vi "st_Wilcoxon diff test.vi"(6 "alternative hypothesis":i32(ring) items=["mean(pop) != mean"=0, "mean(pop) > mean"=1, "mean(pop) < mean"=-1], 9 "significance level":dbl=0.05, 11 "Xi - Yi":dbl[](array[numeric])) -> (0 "error":i32, 2 "p value":dbl, 3 "reject the null hypothesis":bool)   [LabVIEW 2020, in "NI_Gmath.lvlib"]
uses:
  NI_Gmath.lvlib
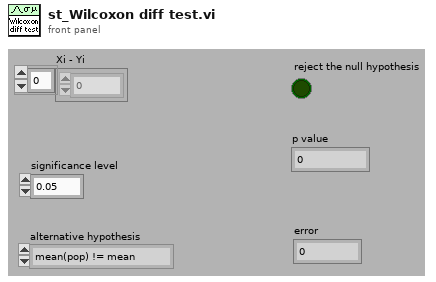
[diagram p1: front panel]
types:
  T1 = cluster{"n":u8, "x min":u8, "x max":u8, "P{W+ >= x}":sgl[]}[]
  T2 = cluster{"n":u8, "x min":u8, "x max":u8, "P{W+ >= x}":sgl[]}
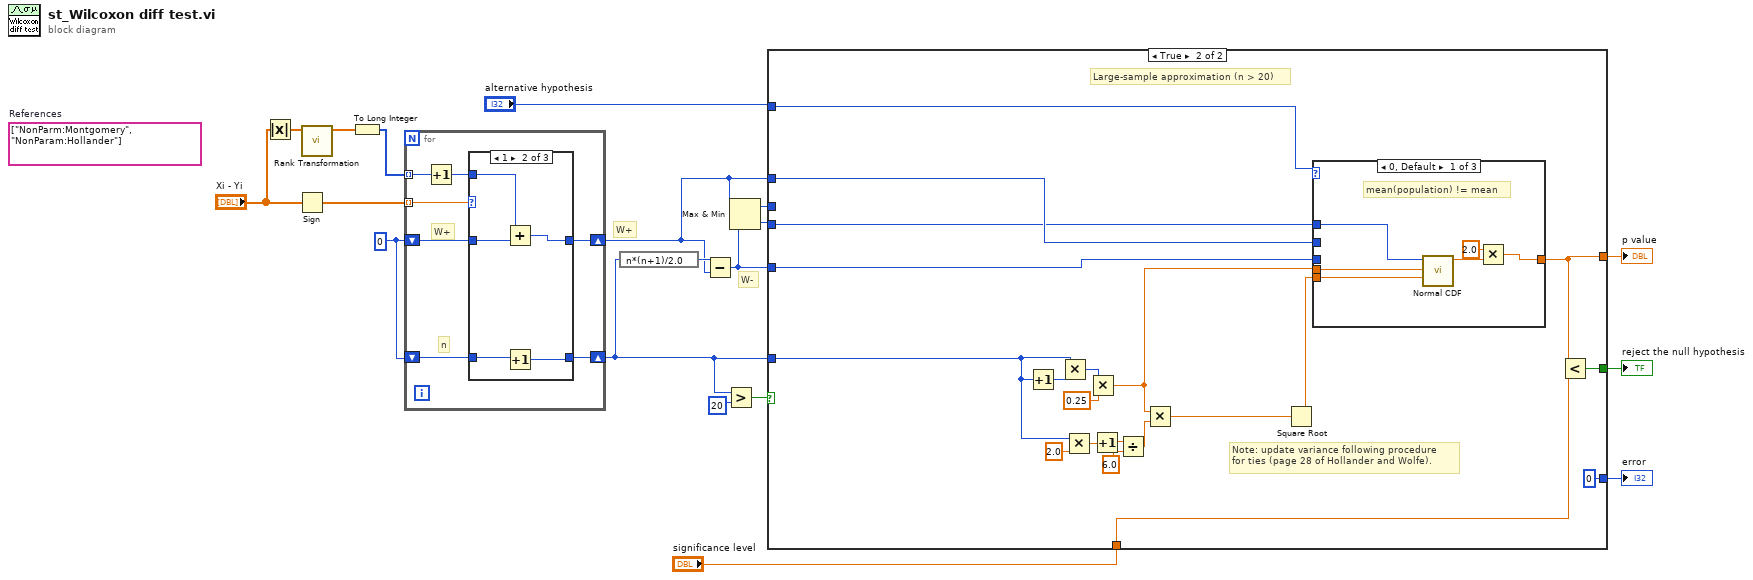
[diagram p0: block diagram]
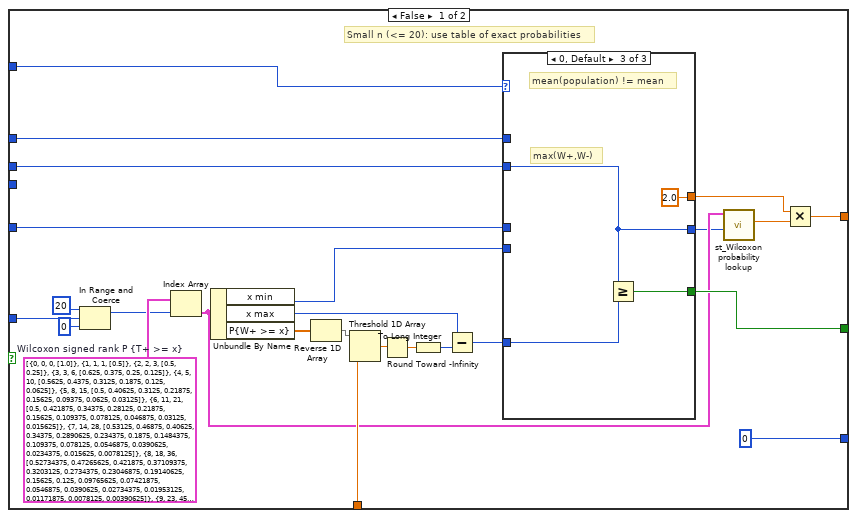
[diagram p2: hidden frame]
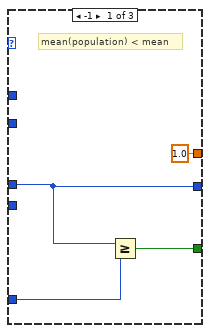
[diagram p3: hidden frame]
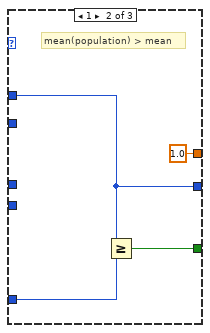
[diagram p4: hidden frame]
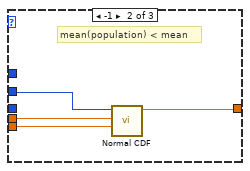
[diagram p5: hidden frame]
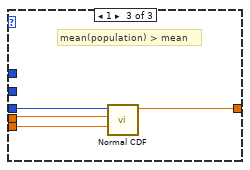
[diagram p6: hidden frame]
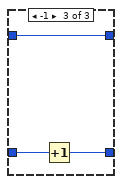
[diagram p8: hidden frame]
diagram:
  (unwired) string[] ["NonParm:Montgomery", "NonParam:Hollander"]  # References
  w13 = 0
  # "W+"
  # "W-"
  n1 = Absolute Value(x="Xi - Yi") -> (abs(x)=w11:dbl[])
  n2 = Sign(1:"Xi - Yi") -> (0:w12:dbl[])
  n3 = call "Rank Transformation.vi"("x"=w11) -> ("rank order x"=w14:dbl[])  [unwired: 9 in, 1 out]
  n4 = To Long Integer(number=w14) -> (32bit integer=w15:i32[])
  n5 = for {
    shift-right: [w25] -> w4
    shift-left: w13 -> [w26]
    tunnel: w12 -> [w24] mode=indexing
    shift-right: [w22] -> w6
    shift-left: w13 -> [w23]
    tunnel: w15 -> [w21] mode=indexing
    # "n"
    # "W+"
    n6 = Increment(x=w21) -> (x+1=w20:i32)
    n7 = case shown="1" w24 {
      tunnel: w26 -> [w28 w33 w36]
      tunnel: [w28 w32 w36] -> w25
      tunnel: [w27 w30 w34] -> w22
      tunnel: w23 -> [w27 w31 w35]
      tunnel: w20 -> [_ w29 _]
      frame 0, Default {
        # "Ties are\nnot counted"
      }
      frame 1 {
        n8 = Add(x=w29, y=w33) -> (x+y=w32:i32)
        n9 = Increment(x=w31) -> (x+1=w30:i32)
      }
      frame -1 {
        n10 = Increment(x=w35) -> (x+1=w34:i32)
      }
    }
  }
  n11 = expression code="n*(n+1)/2.0"(w6) -> (w5:i32)
  n12 = Subtract(x=w5, y=w4) -> (x-y=w3:i32)
  n13 = Greater?(x=w6, y=20) -> (0:w1:bool)
  n14 = Max & Min(x=w4, y=w3) -> (max(x,y)=w2:i32, min(x,y)=w17:i32)
  n15 = case shown="True" w1 {
    tunnel: "alternative hypothesis" -> [w60 w93]
    tunnel: [w37 w92] -> w8
    tunnel: [w50 w91] -> w9
    tunnel: [0 ("error") 0 ("error")] -> w10
    tunnel: w6 -> [w57 w85]
    tunnel: w4 -> [w48 w79]
    tunnel: w3 -> [w47 w78]
    tunnel: "significance level" -> [w56 w75]
    tunnel: w17 -> [_ w74]
    tunnel: w2 -> [w40 _]
    frame False {
      w54 = T1 [{"n"=0, "x min"=0, "x max"=0, "P{W+ >= x}"=[1.0]}, {"n"=1, "x min"=1, "x max"=1, "P{W+ >= x}"=[0.5]}, {"n"=2, "x min"=2, "x max"=3, "P{W+ >= x}"=[0.5, 0.25]}, {"n"=3, "x min"=3, "x max"=6, "P{W+ >= x}"=[0.625, 0.375, 0.25, 0.125]}, {"n"=4, "x min"=5, "x max"=10, "P{W+ >= x}"=[0.5625, 0.4375, 0.3125, 0.1875, 0.125, 0.0625]}, {"n"=5, "x min"=8, "x max"=15, "P{W+ >= x}"=[0.5, 0.40625, 0.3125, 0.21875, 0.15625, 0.09375, 0.0625, 0.03125]}, {"n"=6, "x min"=11, "x max"=21, "P{W+ >= x}"=[0.5, 0.421875, 0.34375, 0.28125, 0.21875, 0.15625, 0.109375, 0.078125, 0.046875, 0.03125, 0.015625]}, {"n"=7, "x min"=14, "x max"=28, "P{W+ >= x}"=[0.53125, 0.46875, 0.40625, 0.34375, 0.2890625, 0.234375, 0.1875, 0.1484375, 0.109375, 0.078125, 0.0546875, 0.0390625, 0.0234375, 0.015625, 0.0078125]}, {"n"=8, "x min"=18, "x max"=36, "P{W+ >= x}"=[0.52734375, 0.47265625, 0.421875, 0.37109375, 0.3203125, 0.2734375, 0.23046875, 0.19140625, 0.15625, 0.125, 0.09765625, 0.07421875, 0.0546875, 0.0390625, 0.02734375, 0.01953125, 0.01171875, 0.0078125, 0.00390625]}, {"n"=9, "x min"=23, "x max"=45, "P{W+ >= x}"=[0.5, 0.45507812, 0.41015625, 0.3671875, 0.32617188, 0.28515625, 0.24804688, 0.21289062, 0.1796875, 0.15039062, 0.125, 0.1015625, 0.08203125, 0.064453125, 0.048828125, 0.037109375, 0.02734375, 0.01953125, 0.013671875, 0.009765625, 0.005859375, 0.00390625, 0.001953125]}, {"n"=10, "x min"=28, "x max"=55, "P{W+ >= x}"=[0.5, 0.4609375, 0.42285156, 0.38476562, 0.34765625, 0.3125, 0.2783203, 0.24609375, 0.21582031, 0.1875, 0.16113281, 0.13769531, 0.11621094, 0.09667969, 0.080078125, 0.06542969, 0.052734375, 0.041992188, 0.032226562, 0.024414062, 0.018554688, 0.013671875, 0.009765625, 0.0068359375, 0.0048828125, 0.0029296875, 0.001953125, 0.0009765625]}, {"n"=11, "x min"=33, "x max"=66, "P{W+ >= x}"=[0.51708984, 0.48291016, 0.44921875, 0.41552734, 0.38232422, 0.35009766, 0.31884766, 0.28857422, 0.25976562, 0.23242188, 0.20654297, 0.18261719, 0.16015625, 0.13916016, 0.12011719, 0.103027344, 0.087402344, 0.07373047, 0.061523438, 0.05078125, 0.041503906, 0.033691406, 0.026855469, 0.020996094, 0.016113281, 0.012207031, 0.009277344, 0.0068359375, 0.0048828125, 0.0034179688, 0.0024414062, 0.0014648438, 0.0009765625, 0.00048828125]}, {"n"=12, "x min"=39, "x max"=78, "P{W+ >= x}"=[0.5151367, 0.48486328, 0.45483398, 0.42504883, 0.3955078, 0.36669922, 0.33862305, 0.31103516, 0.28466797, 0.25927734, 0.23486328, 0.21191406, 0.19018555, 0.16967773, 0.15063477, 0.13305664, 0.11669922, 0.10180664, 0.088134766, 0.075683594, 0.064697266, 0.05493164, 0.046142578, 0.03857422, 0.031982422, 0.026123047, 0.021240234, 0.017089844, 0.013427734, 0.010498047, 0.008056641, 0.0061035156, 0.004638672, 0.0034179688, 0.0024414062, 0.0017089844, 0.0012207031, 0.0007324219, 0.00048828125, 0.00024414062]}, {"n"=13, "x min"=46, "x max"=91, "P{W+ >= x}"=[0.5, 0.47302246, 0.44628906, 0.41967773, 0.39343262, 0.36767578, 0.34240723, 0.31774902, 0.2939453, 0.27087402, 0.24865723, 0.22741699, 0.20715332, 0.18786621, 0.1697998, 0.15270996, 0.13671875, 0.12194824, 0.1081543, 0.095458984, 0.083862305, 0.07324219, 0.06359863, 0.05493164, 0.04711914, 0.040161133, 0.034057617, 0.028686523, 0.023925781, 0.019897461, 0.016357422, 0.013305664, 0.0107421875, 0.008544922, 0.006713867, 0.0052490234, 0.0040283203, 0.0030517578, 0.002319336, 0.0017089844, 0.0012207031, 0.0008544922, 0.00061035156, 0.00036621094, 0.00024414062, 0.00012207031]}, {"n"=14, "x min"=53, "x max"=105, "P{W+ >= x}"=[0.5, 0.47576904, 0.45159912, 0.4276123, 0.40386963, 0.38043213, 0.35742188, 0.3348999, 0.3128662, 0.2915039, 0.270813, 0.25079346, 0.23156738, 0.21313477, 0.1954956, 0.17877197, 0.16290283, 0.14788818, 0.13378906, 0.12060547, 0.10827637, 0.09686279, 0.08630371, 0.076538086, 0.06762695, 0.059448242, 0.052001953, 0.045288086, 0.039245605, 0.033813477, 0.0289917, 0.024719238, 0.020935059, 0.01763916, 0.014770508, 0.012268066, 0.010131836, 0.008300781, 0.006713867, 0.0053710938, 0.004272461, 0.0033569336, 0.0026245117, 0.0020141602, 0.0015258789, 0.001159668, 0.0008544922, 0.00061035156, 0.0004272461, 0.00030517578, 0.00018310547, 0.00012207031, 6.1035156e-05]}, {"n"=15, "x min"=60, "x max"=120, "P{W+ >= x}"=[0.51101685, 0.48898315, 0.46704102, 0.44519043, 0.4234619, 0.40197754, 0.38076782, 0.35986328, 0.339386, 0.31933594, 0.29974365, 0.28070068, 0.26223755, 0.24435425, 0.22714233, 0.2106018, 0.19470215, 0.17956543, 0.16513062, 0.1513977, 0.13842773, 0.12619019, 0.11465454, 0.103881836, 0.093811035, 0.08441162, 0.07571411, 0.06768799, 0.060272217, 0.053497314, 0.047302246, 0.041625977, 0.036499023, 0.03186035, 0.027679443, 0.023956299, 0.020629883, 0.017669678, 0.015075684, 0.012786865, 0.010772705, 0.009033203, 0.007537842, 0.006225586, 0.005126953, 0.004180908, 0.0033569336, 0.0026855469, 0.0021362305, 0.0016784668, 0.0013122559, 0.0010070801, 0.00076293945, 0.000579834, 0.0004272461, 0.00030517578, 0.00021362305, 0.00015258789, 9.1552734e-05, 6.1035156e-05, 3.0517578e-05]}, {"n"=16, "x min"=68, "x max"=136, "P{W+ >= x}"=[0.510025, 0.48997498, 0.4699402, 0.44996643, 0.43013, 0.41044617, 0.39097595, 0.3717804, 0.3528595, 0.3342743, 0.31608582, 0.29829407, 0.28094482, 0.26408386, 0.24771118, 0.23187256, 0.21659851, 0.20187378, 0.18772888, 0.17419434, 0.16125488, 0.14892578, 0.13722229, 0.12611389, 0.115600586, 0.10571289, 0.09640503, 0.087677, 0.07952881, 0.07192993, 0.06486511, 0.05833435, 0.05229187, 0.046722412, 0.041625977, 0.036956787, 0.032699585, 0.028839111, 0.02532959, 0.022155762, 0.019317627, 0.01676941, 0.01449585, 0.012481689, 0.010696411, 0.009124756, 0.007751465, 0.0065460205, 0.005493164, 0.0045928955, 0.0038146973, 0.0031433105, 0.0025787354, 0.002090454, 0.0016784668, 0.0013427734, 0.0010681152, 0.0008392334, 0.00065612793, 0.00050354004, 0.00038146973, 0.000289917, 0.00021362305, 0.00015258789, 0.00010681152, 7.6293945e-05, 4.5776367e-05, 3.0517578e-05, 1.5258789e-05]}, {"n"=17, "x min"=77, "x max"=153, "P{W+ >= x}"=[0.5, 0.48161316, 0.46325684, 0.44498444, 0.42681885, 0.4087906, 0.39095306, 0.37332916, 0.3559494, 0.33885193, 0.32206726, 0.30561066, 0.2895279, 0.27383423, 0.25854492, 0.24369049, 0.2292862, 0.21533966, 0.20188141, 0.18891144, 0.17643738, 0.16447449, 0.15302277, 0.14208221, 0.13166046, 0.12174988, 0.112342834, 0.10344696, 0.095047, 0.087127686, 0.079689026, 0.07271576, 0.066185, 0.06010437, 0.05444336, 0.049186707, 0.044326782, 0.0398407, 0.035705566, 0.031913757, 0.028442383, 0.025268555, 0.022384644, 0.019767761, 0.01739502, 0.015258789, 0.013336182, 0.0116119385, 0.01007843, 0.008712769, 0.007499695, 0.0064315796, 0.005493164, 0.0046691895, 0.0039520264, 0.003326416, 0.002784729, 0.002319336, 0.0019226074, 0.0015792847, 0.0012893677, 0.001045227, 0.0008392334, 0.0006713867, 0.0005340576, 0.0004196167, 0.00032806396, 0.00025177002, 0.00019073486, 0.0001449585, 0.00010681152, 7.6293945e-05, 5.340576e-05, 3.8146973e-05, 2.2888184e-05, 1.5258789e-05, 7.6293945e-06]}, {"n"=18, "x min"=86, "x max"=171, "P{W+ >= x}"=[0.5, 0.48305893, 0.46614075, 0.4492874, 0.43252182, 0.41586304, 0.39935303, 0.38301468, 0.36686325, 0.3509407, 0.3352623, 0.3198471, 0.30472946, 0.2899208, 0.2754364, 0.26130676, 0.24753952, 0.23414612, 0.22114944, 0.20855713, 0.19636917, 0.18460846, 0.173275, 0.16236496, 0.15189743, 0.14186478, 0.13226318, 0.123104095, 0.11437607, 0.10607147, 0.09819412, 0.090732574, 0.083675385, 0.07702255, 0.07075882, 0.06486893, 0.059352875, 0.05419159, 0.049369812, 0.044883728, 0.040714264, 0.036842346, 0.033267975, 0.029968262, 0.026927948, 0.024139404, 0.021583557, 0.019245148, 0.017116547, 0.015182495, 0.01342392, 0.011837006, 0.010406494, 0.009117126, 0.007965088, 0.0069351196, 0.0060157776, 0.005203247, 0.0044822693, 0.0038452148, 0.003288269, 0.0027999878, 0.0023727417, 0.002002716, 0.0016822815, 0.0014038086, 0.0011672974, 0.0009651184, 0.00078964233, 0.00064468384, 0.0005226135, 0.0004196167, 0.00033569336, 0.0002670288, 0.00020980835, 0.00016403198, 0.00012588501, 9.536743e-05, 7.247925e-05, 5.340576e-05, 3.8146973e-05, 2.670288e-05, 1.9073486e-05, 1.1444092e-05, 7.6293945e-06, 3.8146973e-06]}, {"n"=19, "x min"=95, "x max"=190, "P{W+ >= x}"=[0.5078392, 0.4921608, 0.47649193, 0.4608574, 0.4452839, 0.42978668, 0.41439247, 0.39912605, 0.3840027, 0.36904526, 0.35427856, 0.33971405, 0.3253746, 0.3112812, 0.2974434, 0.28388023, 0.2706089, 0.25763893, 0.24498367, 0.23265839, 0.22066689, 0.20902061, 0.19773102, 0.1867981, 0.17622948, 0.16603279, 0.15620422, 0.1467495, 0.13767052, 0.12896347, 0.12062645, 0.11266136, 0.10505867, 0.09781647, 0.090932846, 0.08439636, 0.078201294, 0.07234383, 0.06681061, 0.06159401, 0.05668831, 0.052078247, 0.047756195, 0.043714523, 0.039937973, 0.036417007, 0.033143997, 0.030103683, 0.02728653, 0.024682999, 0.02227974, 0.020065308, 0.018033981, 0.016170502, 0.014465332, 0.012910843, 0.011493683, 0.0102062225, 0.0090408325, 0.007986069, 0.0070343018, 0.0061798096, 0.0054130554, 0.00472641, 0.0041160583, 0.003572464, 0.0030899048, 0.002664566, 0.0022888184, 0.001958847, 0.0016708374, 0.0014190674, 0.0011997223, 0.0010108948, 0.0008468628, 0.000705719, 0.00058555603, 0.0004825592, 0.00039482117, 0.00032234192, 0.00026130676, 0.00020980835, 0.00016784668, 0.0001335144, 0.000104904175, 8.201599e-05, 6.2942505e-05, 4.7683716e-05, 3.6239624e-05, 2.670288e-05, 1.9073486e-05, 1.335144e-05, 9.536743e-06, 5.722046e-06, 3.8146973e-06, 1.9073486e-06]}, {"n"=20, "x min"=105, "x max"=210, "P{W+ >= x}"=[0.50728226, 0.49271774, 0.47816467, 0.46363926, 0.44915867, 0.43474388, 0.4204111, 0.40617752, 0.39206314, 0.37808323, 0.36425304, 0.3505907, 0.33711147, 0.32382774, 0.31075668, 0.29790974, 0.28529835, 0.27293777, 0.2608366, 0.24900436, 0.2374525, 0.2261877, 0.21521664, 0.20454884, 0.19418812, 0.1841383, 0.1744051, 0.16499138, 0.15589714, 0.1471262, 0.1386776, 0.13054943, 0.12274361, 0.11525631, 0.108083725, 0.1012249, 0.09467411, 0.08842659, 0.08247852, 0.076823235, 0.071453094, 0.066363335, 0.061546326, 0.056993484, 0.05269909, 0.048653603, 0.04484749, 0.041275024, 0.03792572, 0.03479004, 0.031861305, 0.029129028, 0.026584625, 0.024220467, 0.022027016, 0.019994736, 0.018116951, 0.016384125, 0.014787674, 0.013320923, 0.011975288, 0.0107421875, 0.009616852, 0.008590698, 0.0076560974, 0.006808281, 0.0060396194, 0.005344391, 0.004717827, 0.0041542053, 0.0036478043, 0.003194809, 0.002790451, 0.0024299622, 0.0021104813, 0.00182724, 0.0015764236, 0.0013561249, 0.001162529, 0.000992775, 0.00084495544, 0.0007162094, 0.0006046295, 0.0005083084, 0.00042533875, 0.00035381317, 0.00029277802, 0.0002412796, 0.00019741058, 0.00016117096, 0.00013065338, 0.000104904175, 8.392334e-05, 6.67572e-05, 5.2452087e-05, 4.1007996e-05, 3.1471252e-05, 2.3841858e-05, 1.8119812e-05, 1.335144e-05, 9.536743e-06, 6.67572e-06, 4.7683716e-06, 2.861023e-06, 1.9073486e-06, 9.536743e-07]}]  # Wilcoxon signed rank P {T+ >= x}
      # "Small n (<= 20): use table of exact probabilities"
      n16 = In Range and Coerce(upper limit=20, x=w57, lower limit=0) -> (coerced(x)=w53:i32)  [unwired: 1 out]
      n17 = Index Array(array=w54, index=w53) -> (element=w42:T2)
      n18 = Unbundle By Name(w42) -> ("x min"=w49:u8, "x max"=w45:u8, "P{W+ >= x}"=w43:sgl[])
      n19 = Reverse 1D Array(array=w43) -> (reversed array=w55:sgl[])
      n20 = Threshold 1D Array(2:w56, 3:w55) -> (0:w52:sgl)  [unwired: 1 in]
      n21 = Round Toward -Infinity(1:w52) -> (0:w51:sgl)
      n22 = To Long Integer(number=w51) -> (32bit integer=w46:i32)
      n23 = Subtract(x=w45, y=w46) -> (x-y=w44:i32)
      n24 = case shown="0, Default" w60 {
        tunnel: w48 -> [_ w67 _]
        tunnel: w44 -> [w64 w69 w73]
        tunnel: [w65 w68 w72] -> w50
        tunnel: w49 -> [_ _ _]
        tunnel: [w63 w67 w71] -> w41
        tunnel: w47 -> [w63 _ _]
        tunnel: w40 -> [_ _ w71]
        tunnel: [1.0 ("x") 1.0 ("x") 2.0 ("x")] -> w38
        frame -1 {
          # "mean(population) < mean"
          n25 = Greater Or Equal?(x=w63, y=w64) -> (x >= y?=w65:bool)
        }
        frame 1 {
          # "mean(population) > mean"
          n26 = Greater Or Equal?(x=w67, y=w69) -> (x >= y?=w68:bool)
        }
        frame 0, Default {
          # "max(W+,W-)"
          # "mean(population) != mean"
          n27 = Greater Or Equal?(x=w71, y=w73) -> (x >= y?=w72:bool)
        }
      }
      n28 = call "st_Wilcoxon probability lookup.vi"("x"=w41, "table column"=w42) -> ("P{W+ >= x}"=w39:dbl)  [unwired: 9 in]
      n29 = Multiply(x=w38, y=w39) -> (x*y=w37:dbl)
    }
    frame True {
      # "Note: update variance following procedure\nfor ties (page 28 of Hollander and Wolfe)."
      # "Large-sample approximation (n > 20)"
      n30 = Increment(x=w85) -> (x+1=w89:i32)
      n31 = Multiply(x=w89, y=w85) -> (x*y=w87:i32)
      n32 = Multiply(x=w85, y=2.0) -> (x*y=w84:dbl)
      n33 = Multiply(x=w87, y=0.25) -> (x*y=w77:dbl)
      n34 = Increment(x=w84) -> (x+1=w83:dbl)
      n35 = Divide(x=w83, y=6.0) -> (x/y=w81:dbl)
      n36 = Multiply(x=w77, y=w81) -> (x*y=w80:dbl)
      n37 = Square Root(x=w80) -> (sqrt(x)=w76:dbl)
      n38 = case shown="0, Default" w93 {
        tunnel: [w95 w101 w104] -> w92
        tunnel: w76 -> [w99 w102 w106]
        tunnel: w77 -> [w98 w103 w107]
        tunnel: w79 -> [_ w100 _]
        tunnel: w78 -> [_ _ w105]
        tunnel: w74 -> [w96 _ _]
        frame 0, Default {
          # "mean(population) != mean"
          n39 = call "Normal CDF.vi"("std"=w99, "mean"=w98, "x"=w96) -> ("cdf(x)"=w97:dbl)  [unwired: 7 in, 1 out]
          n40 = Multiply(x=2.0, y=w97) -> (x*y=w95:dbl)
        }
        frame -1 {
          # "mean(population) < mean"
          n41 = call "Normal CDF.vi"("std"=w102, "mean"=w103, "x"=w100) -> ("cdf(x)"=w101:dbl)  [unwired: 7 in, 1 out]
        }
        frame 1 {
          # "mean(population) > mean"
          n42 = call "Normal CDF.vi"("std"=w106, "mean"=w107, "x"=w105) -> ("cdf(x)"=w104:dbl)  [unwired: 7 in, 1 out]
        }
      }
      n43 = Less?(x=w92, y=w75) -> (x < y?=w91:bool)
    }
  }
  "error" <- w10
  "reject the null hypothesis" <- w9
  "p value" <- w8
